vi "Valuta equilibrio termico.vi"(6 "Valuta tutti i campioni?":bool, 8 "Variazione T eqil term (°C)":dbl, 9 "Tempo equilibrio termico (min)":dbl format="%#_13g", 10 "Array Dt":dbl[](array[numeric]), 11 "Array Time":dbl[](array[numeric])) -> (2 "Equilibrio termico":bool)   [LabVIEW 2019]
uses:
  Global Gestione stop se eq termico.vi
panel:
  out "subarray":dbl[](array[numeric])
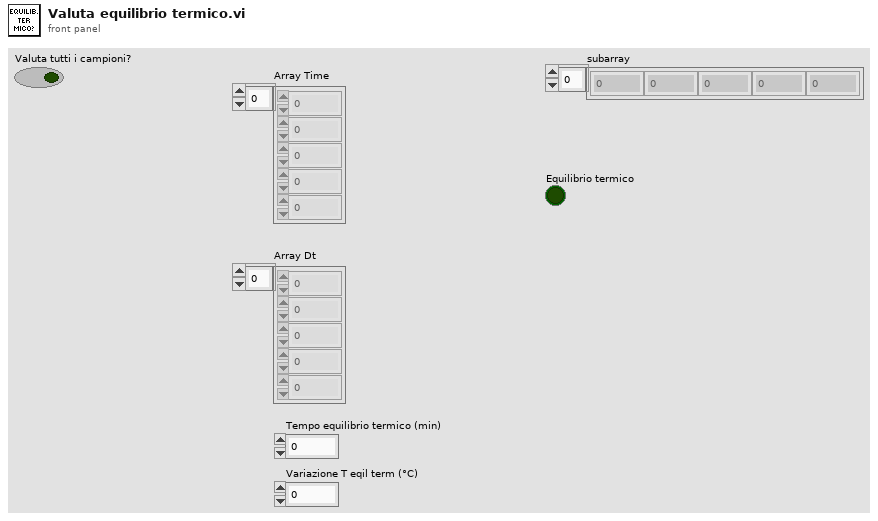
[diagram p1: front panel]
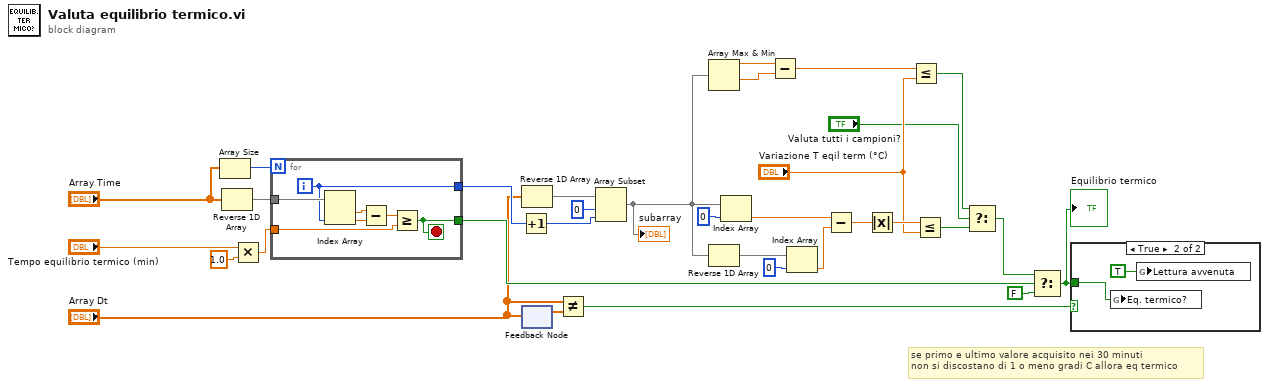
[diagram p0: block diagram]
diagram:
  # "se primo e ultimo valore acquisito nei 30 minuti\nnon si discostano di 1 o meno gradi C allora eq termico"
  n1 = Array Size(array="Array Time") -> (size(s)=w30:i32)
  n2 = Reverse 1D Array(array="Array Time") -> (reversed array=w32:dbl[])
  n3 = Multiply(x="Tempo equilibrio termico (min)", y=1.0) -> (x*y=w20:dbl)
  n4 = for {
    N: w30 -> [_]
    tunnel: w32 -> [w39]
    tunnel: w20 -> [w35]
    tunnel: [w34] -> w24
    tunnel: [w33] -> w19
    i -> [w33]
    stop <- w34 stop-if-true
    n5 = Index Array(array=w39, index #2=w33) -> (element #1=w38:dbl, element #2=w37:dbl)  [unwired: 1 in]
    n6 = Subtract(x=w38, y=w37) -> (x-y=w36:dbl)
    n7 = Greater Or Equal?(x=w36, y=w35) -> (x >= y?=w34:bool)
  }
  n8 = Increment(x=w19) -> (x+1=w18:i32)
  n9 = Reverse 1D Array(array="Array Dt") -> (reversed array=w31:dbl[])
  n10 = feedback-in #1("Array Dt") -> ()
  n11 = feedback #1() -> (w3:dbl[])  [unwired: 1 in]
  n12 = Not Equal?(x="Array Dt", y=w3) -> (x != y?=w2:bool)
  n13 = Array Subset(array=w31, index=0, length=w18) -> (w16:dbl[])
  "subarray" <- w16
  n14 = Array Max & Min(array=w16) -> (max value=w28:dbl, min value=w27:dbl)  [unwired: 2 out]
  n15 = Reverse 1D Array(array=w16) -> (reversed array=w14:dbl[])
  n16 = Index Array(array=w16, index=0) -> (element=w12:dbl)
  n17 = Subtract(x=w28, y=w27) -> (x-y=w26:dbl)
  n18 = Index Array(array=w14, index=0) -> (element=w13:dbl)
  n19 = Subtract(x=w12, y=w13) -> (x-y=w11:dbl)
  n20 = Absolute Value(x=w11) -> (abs(x)=w10:dbl)
  n21 = Less Or Equal?(x=w26, y="Variazione T eqil term (°C)") -> (x <= y?=w8:bool)
  n22 = Less Or Equal?(x=w10, y="Variazione T eqil term (°C)") -> (x <= y?=w7:bool)
  n23 = Select(t=w8, s="Valuta tutti i campioni?", f=w7) -> (s? t:f=w6:bool)
  n24 = Select(t=w6, s=w24, f=FALSE) -> (s? t:f=w1:bool)
  "Equilibrio termico" <- w1
  n25 = case shown="True" w2 {
    tunnel: w1 -> [_ w40]
    frame False {
    }
    frame True {
      n26 = global write "Global Gestione stop se eq termico.vi" "Eq. termico?"(w40) -> ()
      n27 = global write "Global Gestione stop se eq termico.vi" "Lettura avvenuta"(TRUE ("Lettura avvenuta")) -> ()
    }
  }
